vi "Part 1.vi"(11 "Input":string) -> (3 "Output":i64)   [LabVIEW 2021]
uses:
  9d0e809e-66fd-4383-90de-11f2d849ca55.vi
  <userlib>/_OpenG.lib/string/string.llb/Convert EOLs (String)__ogtk.vi
  <vilib>/Comparison/Less/Less Functor/Less Functor.lvclass
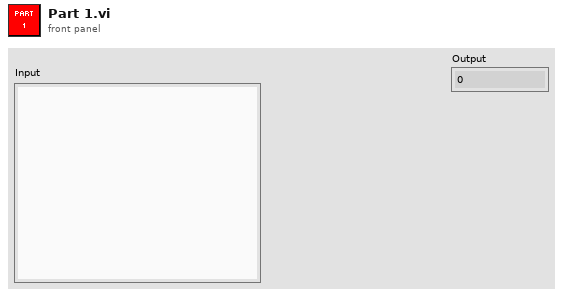
[diagram p1: front panel]
types:
  T1 = cluster{"Type":enum16{"High card", "One pair", "Two pair", "Three of a kind", "Full house", "Four of a kind", "Five of a kind"}, "Hand":string, "Bid":i64}
  T2 = enum16{"High card", "One pair", "Two pair", "Three of a kind", "Full house", "Four of a kind", "Five of a kind"}
  T3 = cluster{"Type":enum16{"High card", "One pair", "Two pair", "Three of a kind", "Full house", "Four of a kind", "Five of a kind"}, "Hand":string, "Bid":i64}[]
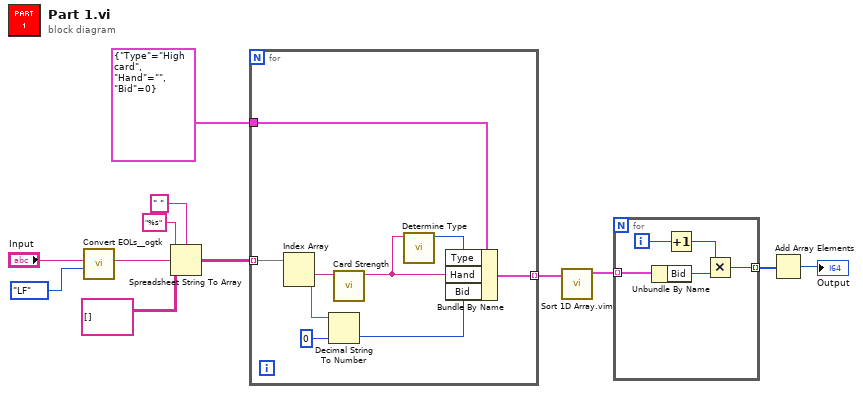
[diagram p0: block diagram]
diagram:
  n1 = call-poly <userlib>:"Convert EOLs__ogtk.vi"("Convert to:"=enum16{"CR", "LF", "CRLF"}."LF", "String in"="Input") -> ("String out"=w8:string)  [unwired: 9 in]
  n2 = Spreadsheet String To Array(delimiter (Tab)=" ", format string="%s", spreadsheet string=w8, array type (2D Dbl)=string[][] []) -> (array=w6:string[][])
  n3 = for {
    tunnel: w6 -> [w21] mode=indexing
    tunnel: T1 {"Type"=enum."High card", "Hand"="", "Bid"=0} ("output cluster") -> [w17]
    tunnel: [w18] -> w5 mode=indexing
    n4 = Index Array(array=w21) -> (element #1=w14:string, element #2=w20:string)  [unwired: 2 in]
    n5 = Decimal String To Number(string=w20, default (0L)=i64 0) -> (number=w15:i64)  [unwired: 1 in, 1 out]
    n6 = call "Card Strength.vi"("Hand In"=w14) -> ("Hand Out"=w13:string)  [unwired: 10 in]
    n7 = call "Determine Type.vi"("Hand"=w13) -> ("Type"=w16:T2)  [unwired: 10 in]
    n8 = Bundle By Name(cluster=w17, "Type"=w16, "Hand"=w13, "Bid"=w15) -> (w18:T1)
  }
  n9 = call "Sort 1D Array.vim"("unsorted array"=w5) -> ("sorted array"=w4:T3)  [unwired: 10 in]
  n10 = for {
    tunnel: w4 -> [w26] mode=indexing
    tunnel: [w22] -> w2 mode=indexing
    i -> [w25]
    n11 = Unbundle By Name(w26) -> ("Bid"=w24:i64)
    n12 = Increment(x=w25) -> (x+1=w23:i32)
    n13 = Multiply(x=w23, y=w24) -> (x*y=w22:i64)
  }
  n14 = Add Array Elements(numeric array=w2) -> (sum=→"Output":i64)
